vi "setFrequency.vi"(7 "Channel":string="0", 8 "error in (no error)":errorcluster, 10 "Frequency [Hz]":dbl, 11 "FgenKeysight in":refnum<class "ArbKeysight.lvclass">) -> (0 "error out":errorcluster, 3 "FgenKeysight out":refnum<class "ArbKeysight.lvclass">)   [LabVIEW 2023, in "ArbKeysight.lvclass"]
doc: "<b>Author:</b> Wolfgang\n<b>Description:</b> Set Output Frequency in Hz"
uses:
  ArbKeysight.lvclass
  ArbKeysight.lvclass/ArbKeysight.ctl
  Arb.lvclass
  Driver/Keysight-33500B.lvlib
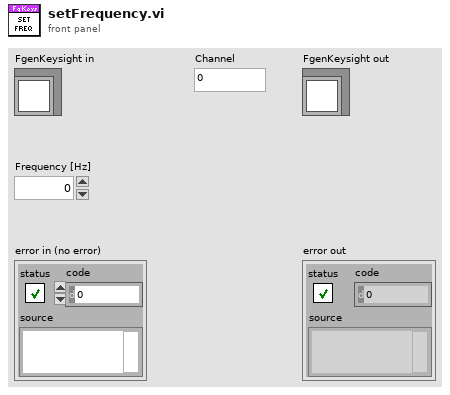
[diagram p1: front panel]
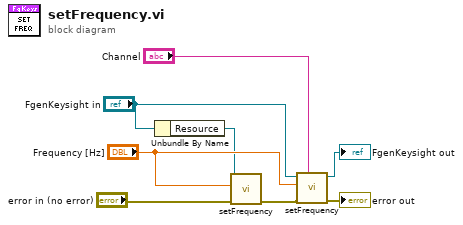
[diagram p0: block diagram]
diagram:
  n1 = Unbundle By Name("FgenKeysight in") -> ("Resource"=w1:refnum<visa-resource-name>)
  n2 = call "setFrequency.vi"("error in (no error)"="error in (no error)", "Frequency"="Frequency [Hz]", "VISA resource name"=w1) -> ("error out"=w5:errorcluster)  [unwired: 7 in, 1 out]
  n3 = call-parent "setFrequency.vi"("Channel"="Channel", "error in (no error)"=w5, "Frequency [Hz]"="Frequency [Hz]", "Fgen in"="FgenKeysight in") -> ("error out"=→"error out":errorcluster, "Fgen out"=→"FgenKeysight out":refnum<class "ArbKeysight.lvclass">)  [unwired: 6 in]
